vi "img_copy.vi"(11 "image in":T1) -> (3 "Image out":T1(plugin-control))   [LabVIEW 2017]
uses:
  <vilib>/vision/Image Controls.llb/IMAQ Image.ctl
  data_loder/data_loader.lvclass
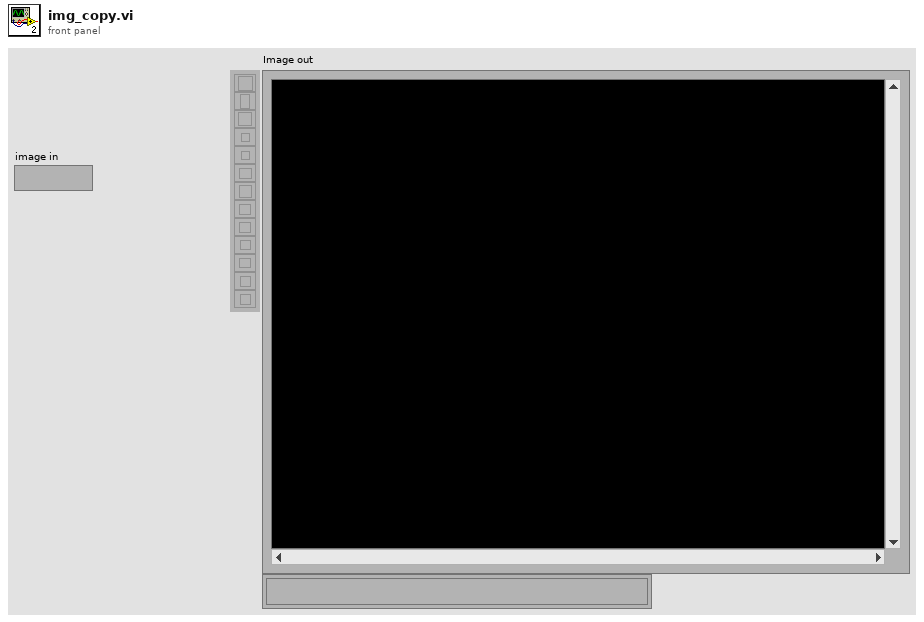
[diagram p1: front panel]
types:
  T1 = typedef "IMAQ Image.ctl" = refnum<image>
  T2 = typedef "Image Type" = u32
  T3 = typedef "imagedata.ctl" = cluster{"image type":i32, "image depth":i32, "image":u8[], "mask":u8[], "colors":u32[], "Rectangle":cluster{"left":i16, "top":i16, "right":i16, "bottom":i16}}
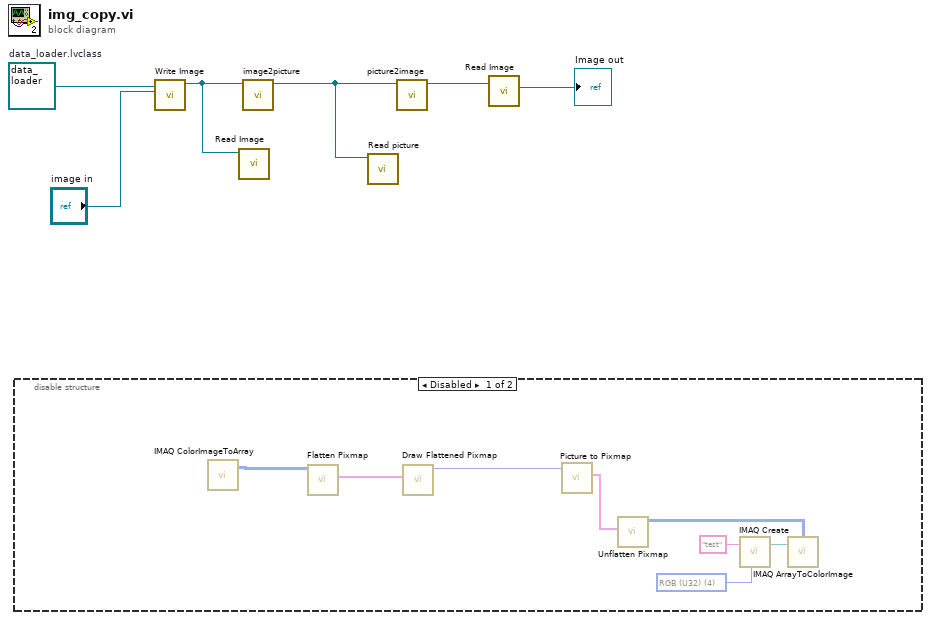
[diagram p0: block diagram]
diagram:
  w5 = refnum<class "data_loader.lvclass"> refnum  # data_loader.lvclass
  n1 = disable-structure shown="Disabled" {
    frame Disabled {
      w12 = T2 4 items=["Grayscale (U8)", "Grayscale (I16)", "Grayscale (SGL)", "Complex (CSG)", "RGB (U32)", "HSL (U32)", "RGB (U64)", "Grayscale (U16)"] ("Image Type")
      n2 = call "IMAQ ColorImageToArray"() -> ("Image Pixels (U32)"=w16:u32[][], "Image"=w8:T1)  [unwired: 3 in, 2 out]
      n3 = call <vilib>:"Flatten Pixmap.vi"("24-bit pixmap"=w16) -> ("image data"=w15:T3)  [unwired: 10 in]
      n4 = call <vilib>:"Draw Flattened Pixmap.vi"("image data"=w15) -> ("new picture"=w9:picture)  [unwired: 8 in]
      n5 = call <vilib>:"Picture to Pixmap.vi"("picture"=w9) -> ("image data"=w10:T3)  [unwired: 9 in, 1 out]
      n6 = call <vilib>:"Unflatten Pixmap.vi"("image data"=w10) -> ("24-bit pixmap"=w11:u32[][])  [unwired: 4 in, 6 out]
      n7 = call "IMAQ Create"("Image Name"="test", "Image Type"=w12) -> ("New Image"=w14:T1)  [unwired: 3 in, 1 out]
      n8 = call "IMAQ ArrayToColorImage"("Image Pixels (U32)"=w11, "Image"=w14) -> ("Image Out"=w7:T1)  [unwired: 3 in, 1 out]
    }
    frame Enabled {
    }
  }
  n9 = call-dynamic "Write Image.vi"("Image"="image in", "data_loader in"=w5) -> ("data_loader out"=w6:refnum<class "data_loader.lvclass">)  [unwired: 8 in, 1 out]
  n10 = call-dynamic "Read Image .vi"("data_loader in"=w6) -> ()  [unwired: 8 in, 3 out]
  n11 = call-dynamic "image2picture.vi"("data_loader in"=w6) -> ("data_loader out"=w1:refnum<class "data_loader.lvclass">)  [unwired: 9 in, 1 out]
  n12 = call-dynamic "Read picture.vi"("data_loader in"=w1) -> ()  [unwired: 8 in, 3 out]
  n13 = call-dynamic "picture2image.vi"("data_loader in"=w1) -> ("data_loader out"=w3:refnum<class "data_loader.lvclass">)  [unwired: 9 in, 1 out]
  n14 = call-dynamic "Read Image .vi"("data_loader in"=w3) -> ("Image"=→"Image out":T1)  [unwired: 8 in, 2 out]
